vi "Friends.vi"() -> ()   [LabVIEW 2020]
uses:
  Test Results/Test Results Base Class.lvclass
panel:
  in  "result":bool
  in  "time/date":timestamp=timestamp(3230114789.968 s since 1904-01-01)
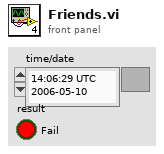
[diagram p1: front panel]
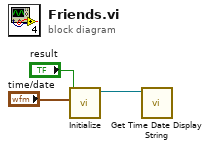
[diagram p0: block diagram]
diagram:
  n1 = call "Initialize.vi"("result"="result", "time/date"="time/date") -> ("Test Results"=w1:refnum<class "Test Results Base Class.lvclass">)  [unwired: 9 in]
  n2 = call "Get Time Date Display String.vi"("test\n results in"=w1) -> ()  [unwired: 8 in, 3 out]
